vi "数据库提取IOT 投入产出时间.vi"() -> (3 "IOT time":T1)   [LabVIEW 2017]
uses:
  IOT time.ctl
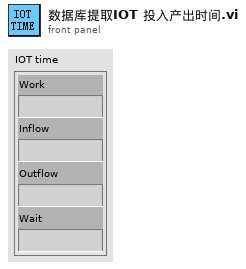
[diagram p1: front panel]
types:
  T1 = typedef "IOT time.ctl" = cluster{"Work":string, "Inflow":string, "Outflow":string, "Wait":string}
  T2 = typedef "动子1&2CT操作选项.ctl" = enum16{"初始化", "出料轴接料", "投掷出料区", "获取寄存器", "更新等待CT"}
  T3 = typedef "动子3&4CT操作选项.ctl" = enum16{"初始化", "扫码+CheckRoute", "BK拍照", "BT+对位", "RT贴合", "Servo压合", "p400复检", "获取寄存器", "更新等待时间"}
  T4 = typedef "上一次缓存.ctl" = cluster{"CT集合":string[], "in /out time":T5, "SN缓存":string}
  T5 = typedef "in_out time.ctl" = cluster{"input-time":string, "output-time":string, "wait-starttime":dbl, "wait-time":string}
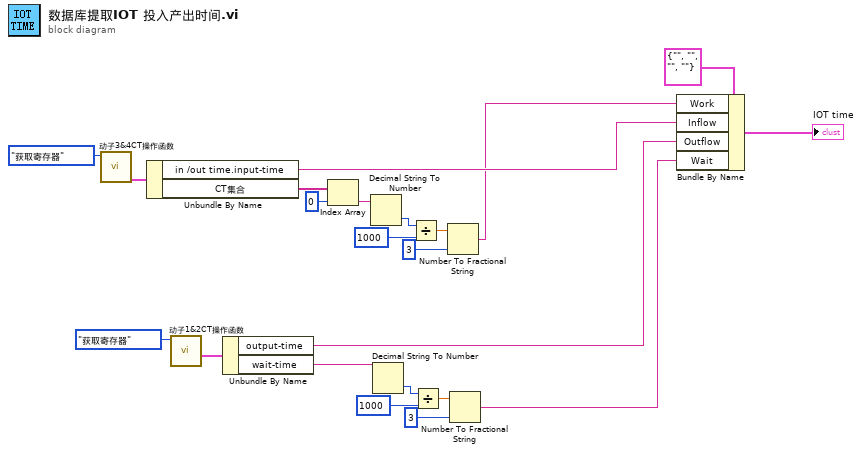
[diagram p0: block diagram]
diagram:
  n1 = call "动子3&4CT操作函数.vi"("CT操作选项"=动子3&4CT操作选项."获取寄存器") -> ("上一次缓存"=w18:T4)  [unwired: 8 in, 2 out]
  n2 = Unbundle By Name(w18) -> ("in /out time.input-time"=w15:string, "CT集合"=w14:string[])
  n3 = call "动子1&2CT操作函数.vi"("CT操作选项"=动子1&2CT操作选项."获取寄存器") -> ("in /out time"=w17:T5)  [unwired: 9 in, 1 out]
  n4 = Unbundle By Name(w17) -> ("output-time"=w16:string, "wait-time"=w2:string)
  n5 = Index Array(array=w14, index=0 ("索引")) -> (element=w12:string)
  n6 = Decimal String To Number(string=w12) -> (number=w11:i32)  [unwired: 2 in, 1 out]
  n7 = Decimal String To Number(string=w2) -> (number=w3:i32)  [unwired: 2 in, 1 out]
  n8 = Divide(x=w11, y=1000) -> (x/y=w9:dbl)
  n9 = Divide(x=w3, y=1000) -> (x/y=w5:dbl)
  n10 = Number To Fractional String(number=w9, precision (6)=i16 3 ("精度(6)")) -> (F-format string=w7:string)  [unwired: 2 in]
  n11 = Number To Fractional String(number=w5, precision (6)=i16 3 ("精度(6)")) -> (F-format string=w1:string)  [unwired: 2 in]
  n12 = Bundle By Name(cluster=T1 {"Work"="", "Inflow"="", "Outflow"="", "Wait"=""} ("IOT time"), "Work"=w7, "Inflow"=w15, "Outflow"=w16, "Wait"=w1) -> (→"IOT time":T1)
